vi "Call Function with Arrays.vi"(8 "error in (no error)":errorcluster) -> (0 "error out":errorcluster)   [LabVIEW 2020]
uses:
  908d8fb0-7b42-46e8-9e96-a0c6d44c2c93.vi
  G-Embedded-Python-Interpreter-Toolkit/Null Py Object Refnum.vi
  908d8fb0-7b42-46e8-9e96-a0c6d44c2c93.vi/96ddca92-7bbf-40e2-a1a5-d32f291eb6af.vi
  G-Embedded-Python-Interpreter-Toolkit/Python Object Reference to Pointer Sized Ref.vi
  G-Embedded-Python-Interpreter-Toolkit/Pointer Sized Ref to Python Object Reference.vi
  G-Embedded-Python-Interpreter-Toolkit/Merge Call Library Errors.vi
  G-Embedded-Python-Interpreter-Toolkit/Generate Argument Type Info.vi
  <vilib>/addons/_JKI Toolkits/Caraya/classes/Assert/Assert Not Error.vi
  <vilib>/addons/_JKI Toolkits/Caraya/classes/Assert/Assert Equal Value and Type_Variant.vi
  G-Embedded-Python-Interpreter-Toolkit/G-Embedded-Python-Interpreter-Toolkit.lvlib
  <vilib>/addons/_JKI Toolkits/Caraya/classes/Test/Test.lvclass
  <vilib>/addons/_JKI Toolkits/Caraya/classes/Assert/Assert.lvclass
panel:
  out "Print Ouptut":string
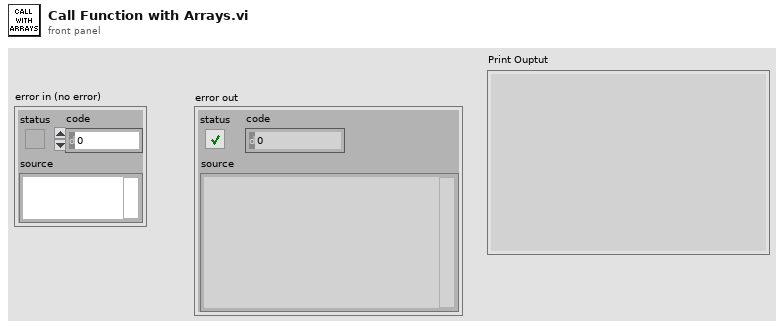
[diagram p1: front panel]
types:
  T1 = typedef "G-Embedded-Python-Interpreter-Toolkit.lvlib/Python Object Reference.ctl" = refnum<k1>
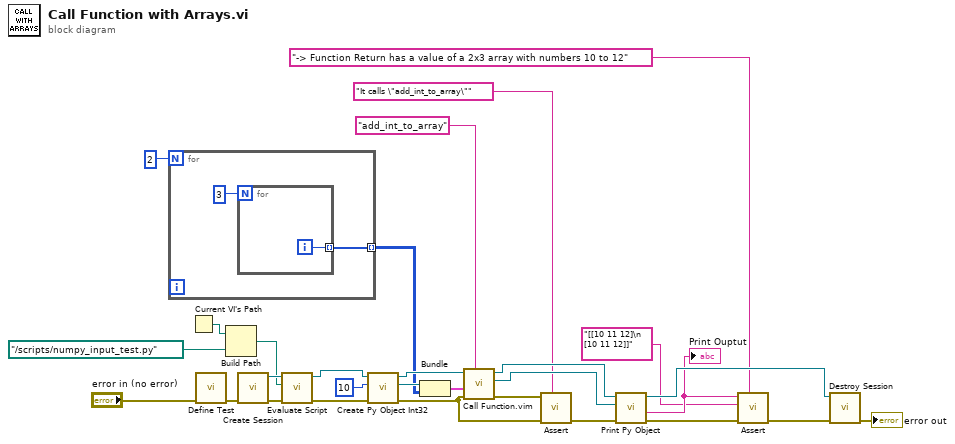
[diagram p0: block diagram]
diagram:
  n1 = for {
    N: 2 -> [_]
    tunnel: [w30] -> w5 mode=indexing
    n2 = for {
      N: 3 -> [_]
      tunnel: [w32] -> w30 mode=indexing
      i -> [w32]
    }
  }
  n3 = Current VI's Path() -> (path=w26:path)
  n4 = call <vilib>:"Define Test.vi"("error in (no error)"="error in (no error)") -> ("error out"=w1:errorcluster)  [unwired: 10 in]
  n5 = Build Path(base path=w26, name or relative path=path "../scripts/numpy_input_test.py" ("Path")) -> (appended path=w24:path)
  n6 = call "Create Session.vi"("error in (no error)"=w1) -> ("error out"=w23:errorcluster, "Session Handle"=w27:refnum<data-value>)  [unwired: 9 in]
  n7 = call "Evaluate Script.vi"("error in (no error)"=w23, "Script File Path"=w24, "Session Handle in"=w27) -> ("error out"=w21:errorcluster, "Session Handle out"=w22:refnum<data-value>)  [unwired: 7 in]
  n8 = call "Create Py Object Int32.vi"("error in (no error)"=w21, "Value"=10, "Session Handle in"=w22) -> ("error out"=w13:errorcluster, "Python Object Refnum"=w6:T1, "Session Handle out"=w20:refnum<data-value>)  [unwired: 6 in]
  n9 = Bundle("Python Object Refnum"=w6, w5) -> (w4:cluster{"Python Object Refnum":T1, i32[][]})  [unwired: 1 in]
  n10 = call "Call Function.vim"("Function Name"="add_int_to_array", "error in (no error)"=w13, "Arguments in (Default - None)"=w4, "Data Value Reference in"=w20) -> ("error out"=w12:errorcluster, "Returned Python Object Refnum"=w18:T1, "Data Value Reference out"=w19:refnum<data-value>)  [unwired: 5 in]
  n11 = call-poly <vilib>:"Assert.vi"("Label"="It calls \"add_int_to_array\"", "error in (no error)"=w13, "Not Error?"=w12) -> ("error out"=w11:errorcluster)  [unwired: 8 in]
  n12 = call "Print Py Object.vi"("error in (no error)"=w11, "Python Object Refnum in"=w18, "Session Handle in"=w19) -> ("error out"=w10:errorcluster, "Print Ouptut"=w3:string, "Session Handle out"=w17:refnum<data-value>)  [unwired: 5 in, 1 out]
  "Print Ouptut" <- w3
  n13 = call-poly <vilib>:"Assert.vi"("Label"="-> Function Return has a value of a 2x3 array with numbers 10 to 12", "error in (no error)"=w10, "Y"="[[10 11 12]\n [10 11 12]]" ("Print Ouptut"), "X"=w3) -> ("error out"=w16:errorcluster)  [unwired: 7 in]
  n14 = call "Destroy Session.vi"("error in (no error)"=w16, "Session Handle"=w17) -> ("error out"=→"error out":errorcluster)  [unwired: 9 in]
